vi "Exit Initialize (User).vi"(8 "error in":errorcluster, 11 "Node in":refnum<class "AMS Power Supply Template.lvclass">) -> (0 "error out":errorcluster, 3 "Node out":refnum<class "AMS Power Supply Template.lvclass">)   [LabVIEW 2023, in "AMS Power Supply Template.lvlib" / "AMS Power Supply Template.lvclass"]
uses:
  AMS Power Supply Template.lvclass
  C:/Program Files/National Instruments/LabVIEW 2024/vi.lib/ADAS Replay HIL/Template Node/Plugin/Template Node/Template Node.lvclass
  <vilib>/ADAS Replay HIL/Template Node/Plugin/Template Node/Template Node.lvclass/Template Node.ctl
  C:/Program Files/National Instruments/AMS plugin/Capabilities/Capabilities/Utilities/Utilities.lvlib
  <vilib>/ADAS Replay HIL/Template Node/Plugin/Template Node/Template Node.lvclass
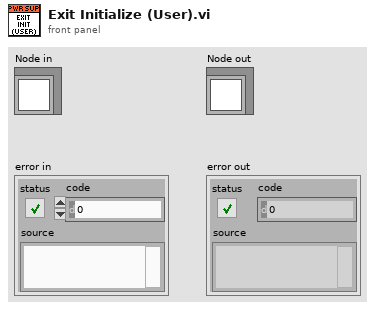
[diagram p1: front panel]
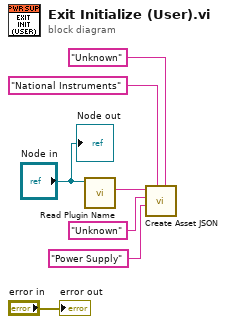
[diagram p0: block diagram]
diagram:
  n1 = call <vilib>:"Read Plugin Name.vi"("Template Node in"="Node in") -> ("Plugin Name"=w7:string)  [unwired: 8 in, 2 out]
  n2 = call "Create Asset JSON.vi"("firmwareVersion"="Unknown", "vendorName"="National Instruments", "modelName"="Power Supply", "serialNumber"="Unknown", "pluginName"=w7) -> ()  [unwired: 5 in, 2 out]
  "Node out" <- "Node in"
  "error out" <- "error in"
